vi "CorrelImages (SubVI)Single.vi"(8 "last drift detected":i32, 9 "Correlate":u16(ring) items=["first Frame", "successive Frames"], 10 "Ref Array":dbl[][](array[numeric]), 11 "New Image":dbl[][](array[numeric])) -> (2 "Y drift":i32, 3 "X drift":i32, 4 "Ref Array out":dbl[][](array[numeric]), 5 "Queue Steps":i32=40)   [LabVIEW 2014]
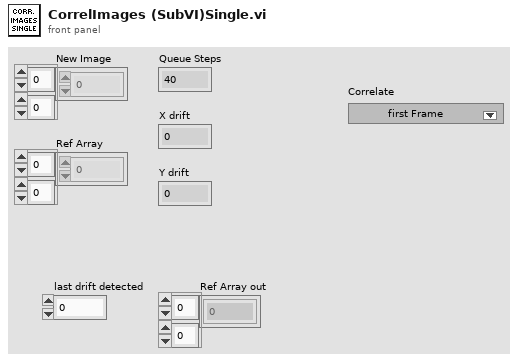
[diagram p1: front panel]
types:
  T1 = enum16{"nothing", "average", "8bit", "average/plane", "minimum", "plane", "average/stddev", "plane/average", "slope"}
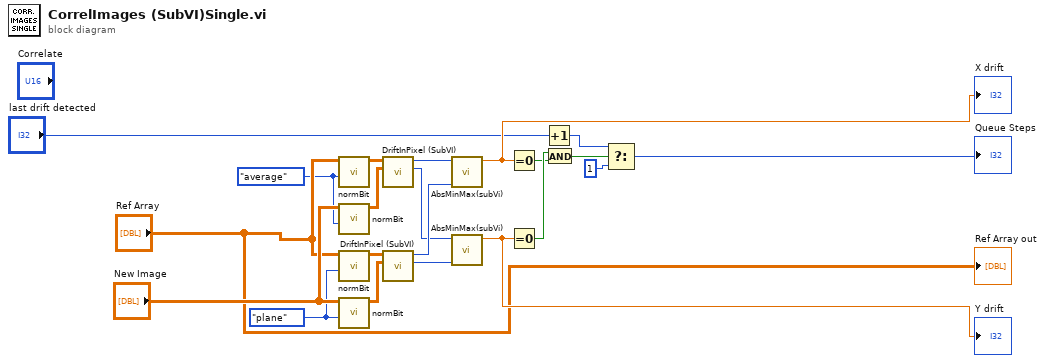
[diagram p0: block diagram]
diagram:
  w5 = T1."plane" ("method")
  w6 = T1."average" ("method")
  n1 = call "normBit.vi"("method"=w6, "Rxy"="Ref Array") -> ("Array"=w7:dbl[][])  [unwired: 8 in, 1 out]
  n2 = call "normBit.vi"("method"=w6, "Rxy"="New Image") -> ("Array"=w10:dbl[][])  [unwired: 8 in, 1 out]
  n3 = call "normBit.vi"("method"=w5, "Rxy"="Ref Array") -> ("Array"=w8:dbl[][])  [unwired: 8 in, 1 out]
  n4 = call "normBit.vi"("method"=w5, "Rxy"="New Image") -> ("Array"=w9:dbl[][])  [unwired: 8 in, 1 out]
  n5 = call "DriftInPixel (SubVI).vi"("New image"=w10, "Ref image"=w7) -> ("Y drift"=w2:i32, "X drift"=w3:i32)  [unwired: 7 in, 1 out]
  n6 = call "DriftInPixel (SubVI).vi"("New image"=w9, "Ref image"=w8) -> ("Y drift"=w1:i32, "X drift"=w4:i32)  [unwired: 7 in, 1 out]
  n7 = call "AbsMinMax(subVi).vi"("y"=w4, "x"=w3) -> ("abs max"=w19:dbl)  [unwired: 8 in, 1 out]
  "X drift" <- w19
  n8 = call "AbsMinMax(subVi).vi"("y"=w1, "x"=w2) -> ("abs max"=w20:dbl)  [unwired: 8 in, 1 out]
  "Y drift" <- w20
  n9 = Equal To 0?(x=w19) -> (x = 0?=w14:bool)
  n10 = Equal To 0?(x=w20) -> (x = 0?=w15:bool)
  n11 = Increment(x="last drift detected") -> (x+1=w11:i32)
  n12 = And(x=w15, y=w14) -> (x .and. y?=w13:bool)
  n13 = Select(t=w11, s=w13, f=1) -> (s? t:f=→"Queue Steps":i32)
  "Ref Array out" <- "Ref Array"
